vi "Remove Group IVI Devices.vi"(9 "IVI Names":string[][](array[string])=[["SNS_A", "SNS_A", "SRC_C", "SRC_C"], ["SNS_A", "SNS_A", "SRC_C", "SRC_C"], ["SNS_A", "SNS_A", "SRC_C", "SRC_C"], ["SNS_A", "SNS_A", "SRC_C", "SRC_C"], ["SNS_A", "SNS_A", "SRC_C", "SRC_C"], ["SNS_A", "SNS_A", "SRC_C", "SRC_C"], ["SNS_A", "SNS_A", "SRC_C", "SRC_C"], ["SNS_A", "SNS_A", "SRC_C", "SRC_C"], ["SNS_A", "SNS_A", "SRC_C", "SRC_C"], ["SNS_A", "SNS_A", "SRC_C", "SRC_C"], ["SNS_A", "SNS_A", "SRC_C", "SRC_C"], ["SNS_A", "SNS_A", "SRC_C", "SRC_C"], ["SNS_A", "SNS_A", "SRC_C", "SRC_C"], ["SNS_A", "SNS_A", "SRC_C", "SRC_C"], ["SNS_A", "SNS_A", "SRC_C", "SRC_C"], ["SNS_A", "SNS_A", "SRC_C", "SRC_C"], ["SNS_A", "SNS_A", "SRC_C", "SRC_C"], ["SNS_A", "SNS_A", "SRC_C", "SRC_C"], ["SNS_A", "SNS_A", "SRC_C", "SRC_C"], ["SNS_A", "SNS_A", "SRC_C", "SRC_C"], ["SNS_A", "SNS_A", "SRC_C", "SRC_C"], ["SNS_A", "SNS_A", "SRC_C", "SRC_C"], ["SNS_A", "SNS_A", "SRC_C", "SRC_C"], ["SNS_A", "SNS_A", "SRC_C", "SRC_C"], ["SNS_A", "SNS_A", "SRC_C", "SRC_C"], ["SNS_A", "SNS_A", "SRC_C", "SRC_C"], ["SNS_A", "SNS_A", "SRC_C", "SRC_C"], ["SNS_A", "SNS_A", "SRC_C", "SRC_C"], ["SNS_A", "SNS_A", "SRC_C", "SRC_C"], ["SNS_A", "SNS_A", "SRC_C", "SRC_C"], ["SNS_A", "SNS_A", "SRC_C", "SRC_C"], ["SNS_A", "SNS_A", "SRC_C", "SRC_C"], ["SNS_A", "SNS_A", "SRC_C", "SRC_C"], ["SNS_A", "SNS_A", "SRC_C", "SRC_C"], ["SNS_A", "SNS_A", "SRC_C", "SRC_C"], ["SNS_A", "SNS_A", "SRC_C", "SRC_C"], ["SNS_A", "SNS_A", "SRC_C", "SRC_C"], ["SNS_A", "SNS_A", "SRC_C", "SRC_C"], ["SNS_A", "SNS_A", "SRC_C", "SRC_C"], ["SNS_A", "SNS_A", "SRC_C", "SRC_C"], ["SNS_A", "SNS_A", "SRC_C", "SRC_C"], ["SNS_A", "SNS_A", "SRC_C", "SRC_C"], ["SNS_A", "SNS_A", "SRC_C", "SRC_C"], ["SNS_A", "SNS_A", "SRC_C", "SRC_C"], ["SNS_A", "SNS_A", "SRC_C", "SRC_C"], ["SNS_A", "SNS_A", "SRC_C", "SRC_C"], ["SNS_A", "SNS_A", "SRC_C", "SRC_C"], ["SNS_A", "SNS_A", "SRC_C", "SRC_C"], ["SNS_A", "SNS_A", "SRC_C", "SRC_C"], ["SNS_A", "SNS_A", "SRC_C", "SRC_C"], ["SNS_A", "SNS_A", "SRC_C", "SRC_C"], ["SNS_A", "SNS_A", "SRC_C", "SRC_C"], ["SNS_A", "SNS_A", "SRC_C", "SRC_C"], ["SNS_A", "SNS_A", "SRC_C", "SRC_C"], ["SNS_A", "SNS_A", "SRC_C", "SRC_C"], ["SNS_A", "SNS_A", "SRC_C", "SRC_C"], ["SNS_A", "SNS_A", "SRC_C", "SRC_C"], ["SNS_A", "SNS_A", "SRC_C", "SRC_C"], ["SNS_A", "SNS_A", "SRC_C", "SRC_C"], ["SNS_A", "SNS_A", "SRC_C", "SRC_C"], ["SNS_A", "SNS_A", "SRC_C", "SRC_C"], ["SNS_A", "SNS_A", "SRC_C", "SRC_C"], ["SNS_A", "SNS_A", "SRC_C", "SRC_C"], ["SNS_A", "SNS_A", "SRC_C", "SRC_C"], ["SNS_A", "SNS_A", "PXI1Slot14", ""], ["SNS_A", "SNS_A", "PXI1Slot14", ""], ["SNS_A", "SNS_A", "PXI1Slot14", ""], ["SNS_A", "SNS_A", "PXI1Slot14", ""], ["SNS_A", "SNS_A", "PXI1Slot14", ""], ["SNS_A", "SNS_A", "PXI1Slot14", ""], ["SNS_A", "SNS_A", "PXI1Slot14", ""], ["SNS_A", "SNS_A", "PXI1Slot14", ""], ["SNS_A", "SNS_A", "PXI1Slot14", ""], ["SNS_A", "SNS_A", "PXI1Slot14", ""], ["SNS_A", "SNS_A", "PXI1Slot14", ""], ["SNS_A", "SNS_A", "PXI1Slot14", ""], ["SNS_A", "SNS_A", "PXI1Slot14", ""], ["SNS_A", "SNS_A", "PXI1Slot14", ""], ["SNS_A", "SNS_A", "PXI1Slot14", ""], ["SNS_A", "SNS_A", "PXI1Slot14", ""], ["SNS_A", "SNS_A", "PXI1Slot14", ""], ["SNS_A", "SNS_A", "PXI1Slot14", ""], ["SNS_A", "SNS_A", "PXI1Slot14", ""], ["SNS_A", "SNS_A", "PXI1Slot14", ""], ["SNS_A", "SNS_A", "PXI1Slot14", ""], ["SNS_A", "SNS_A", "PXI1Slot14", ""], ["SNS_A", "SNS_A", "PXI1Slot14", ""], ["SNS_A", "SNS_A", "PXI1Slot14", ""], ["SNS_A", "SNS_A", "PXI1Slot14", ""], ["SNS_A", "SNS_A", "PXI1Slot14", ""], ["SNS_A", "SNS_A", "PXI1Slot14", ""], ["SNS_A", "SNS_A", "PXI1Slot14", ""], ["SNS_A", "SNS_A", "PXI1Slot14", ""], ["SNS_A", "SNS_A", "PXI1Slot14", ""], ["SNS_A", "SNS_A", "PXI1Slot14", ""], ["SNS_A", "SNS_A", "PXI1Slot14", ""], ["SNS_A", "SNS_A", "PXI1Slot14", ""], ["SNS_A", "SNS_A", "PXI1Slot14", ""], ["SNS_A", "SNS_A", "PXI1Slot14", ""], ["SNS_A", "SNS_A", "PXI1Slot14", ""], ["SNS_A", "SNS_A", "PXI1Slot14", ""], ["SNS_A", "SNS_A", "PXI1Slot14", ""], ["SNS_A", "SNS_A", "PXI1Slot14", ""], ["SNS_A", "SNS_A", "PXI1Slot14", ""], ["SNS_A", "SNS_A", "PXI1Slot14", ""], ["SNS_A", "SNS_A", "PXI1Slot14", ""], ["SNS_A", "SNS_A", "PXI1Slot14", ""], ["SNS_A", "SNS_A", "PXI1Slot14", ""], ["SNS_A", "SNS_A", "PXI1Slot14", ""], ["SNS_A", "SNS_A", "PXI1Slot14", ""], ["SNS_A", "SNS_A", "PXI1Slot14", ""], ["SNS_A", "SNS_A", "PXI1Slot14", ""], ["SNS_A", "SNS_A", "PXI1Slot14", ""], ["SNS_A", "SNS_A", "PXI1Slot14", ""], ["SNS_A", "SNS_A", "PXI1Slot14", ""], ["SNS_A", "SNS_A", "PXI1Slot14", ""], ["SNS_A", "SNS_A", "PXI1Slot14", ""], ["SNS_A", "SNS_A", "PXI1Slot14", ""], ["SNS_A", "SNS_A", "PXI1Slot14", ""], ["SNS_A", "SNS_A", "PXI1Slot14", ""], ["SNS_A", "SNS_A", "PXI1Slot14", ""], ["SNS_A", "SNS_A", "PXI1Slot14", ""], ["SNS_A", "SNS_A", "PXI1Slot14", ""], ["SNS_A", "SNS_A", "PXI1Slot14", ""], ["SNS_A", "SNS_A", "PXI1Slot14", ""], ["SNS_A", "SNS_A", "PXI1Slot14", ""], ["SNS_A", "SNS_A", "PXI1Slot14", ""]], 11 "Specifications":string[][](array[string])=[["Ch0", "[SNS_A/ab2->SNS_A/card1r2->SNS_A/c0]", "[SNS_A/ab3->SNS_A/card1r3->SNS_A/c1]", "[SRC_C/ab0->SRC_C/card1r0->SRC_C/c0]", "[SRC_C/ab1->SRC_C/card1r1->SRC_C/c1]"], ["Ch1", "[SNS_A/ab2->SNS_A/card1r2->SNS_A/c2]", "[SNS_A/ab3->SNS_A/card1r3->SNS_A/c3]", "[SRC_C/ab0->SRC_C/card1r0->SRC_C/c2]", "[SRC_C/ab1->SRC_C/card1r1->SRC_C/c3]"], ["Ch2", "[SNS_A/ab2->SNS_A/card1r2->SNS_A/c4]", "[SNS_A/ab3->SNS_A/card1r3->SNS_A/c5]", "[SRC_C/ab0->SRC_C/card1r0->SRC_C/c4]", "[SRC_C/ab1->SRC_C/card1r1->SRC_C/c5]"], ["Ch3", "[SNS_A/ab2->SNS_A/card1r2->SNS_A/c6]", "[SNS_A/ab3->SNS_A/card1r3->SNS_A/c7]", "[SRC_C/ab0->SRC_C/card1r0->SRC_C/c6]", "[SRC_C/ab1->SRC_C/card1r1->SRC_C/c7]"], ["Ch4", "[SNS_A/ab2->SNS_A/card1r2->SNS_A/c8]", "[SNS_A/ab3->SNS_A/card1r3->SNS_A/c9]", "[SRC_C/ab0->SRC_C/card1r0->SRC_C/c8]", "[SRC_C/ab1->SRC_C/card1r1->SRC_C/c9]"], ["Ch5", "[SNS_A/ab2->SNS_A/card1r2->SNS_A/c10]", "[SNS_A/ab3->SNS_A/card1r3->SNS_A/c11]", "[SRC_C/ab0->SRC_C/card1r0->SRC_C/c10]", "[SRC_C/ab1->SRC_C/card1r1->SRC_C/c11]"], ["Ch6", "[SNS_A/ab2->SNS_A/card1r2->SNS_A/c12]", "[SNS_A/ab3->SNS_A/card1r3->SNS_A/c13]", "[SRC_C/ab0->SRC_C/card1r0->SRC_C/c12]", "[SRC_C/ab1->SRC_C/card1r1->SRC_C/c13]"], ["Ch7", "[SNS_A/ab2->SNS_A/card1r2->SNS_A/c14]", "[SNS_A/ab3->SNS_A/card1r3->SNS_A/c15]", "[SRC_C/ab0->SRC_C/card1r0->SRC_C/c14]", "[SRC_C/ab1->SRC_C/card1r1->SRC_C/c15]"], ["Ch8", "[SNS_A/ab2->SNS_A/card1r2->SNS_A/c16]", "[SNS_A/ab3->SNS_A/card1r3->SNS_A/c17]", "[SRC_C/ab0->SRC_C/card1r0->SRC_C/c16]", "[SRC_C/ab1->SRC_C/card1r1->SRC_C/c17]"], ["Ch9", "[SNS_A/ab2->SNS_A/card1r2->SNS_A/c18]", "[SNS_A/ab3->SNS_A/card1r3->SNS_A/c19]", "[SRC_C/ab0->SRC_C/card1r0->SRC_C/c18]", "[SRC_C/ab1->SRC_C/card1r1->SRC_C/c19]"], ["Ch10", "[SNS_A/ab2->SNS_A/card1r2->SNS_A/c20]", "[SNS_A/ab3->SNS_A/card1r3->SNS_A/c21]", "[SRC_C/ab0->SRC_C/card1r0->SRC_C/c20]", "[SRC_C/ab1->SRC_C/card1r1->SRC_C/c21]"], ["Ch11", "[SNS_A/ab2->SNS_A/card1r2->SNS_A/c22]", "[SNS_A/ab3->SNS_A/card1r3->SNS_A/c23]", "[SRC_C/ab0->SRC_C/card1r0->SRC_C/c22]", "[SRC_C/ab1->SRC_C/card1r1->SRC_C/c23]"], ["Ch12", "[SNS_A/ab2->SNS_A/card1r2->SNS_A/c24]", "[SNS_A/ab3->SNS_A/card1r3->SNS_A/c25]", "[SRC_C/ab0->SRC_C/card1r0->SRC_C/c24]", "[SRC_C/ab1->SRC_C/card1r1->SRC_C/c25]"], ["Ch13", "[SNS_A/ab2->SNS_A/card1r2->SNS_A/c26]", "[SNS_A/ab3->SNS_A/card1r3->SNS_A/c27]", "[SRC_C/ab0->SRC_C/card1r0->SRC_C/c26]", "[SRC_C/ab1->SRC_C/card1r1->SRC_C/c27]"], ["Ch14", "[SNS_A/ab2->SNS_A/card1r2->SNS_A/c28]", "[SNS_A/ab3->SNS_A/card1r3->SNS_A/c29]", "[SRC_C/ab0->SRC_C/card1r0->SRC_C/c28]", "[SRC_C/ab1->SRC_C/card1r1->SRC_C/c29]"], ["Ch15", "[SNS_A/ab2->SNS_A/card1r2->SNS_A/c30]", "[SNS_A/ab3->SNS_A/card1r3->SNS_A/c31]", "[SRC_C/ab0->SRC_C/card1r0->SRC_C/c30]", "[SRC_C/ab1->SRC_C/card1r1->SRC_C/c31]"], ["Ch16", "[SNS_A/ab2->SNS_A/card1r2->SNS_A/c32]", "[SNS_A/ab3->SNS_A/card1r3->SNS_A/c33]", "[SRC_C/ab0->SRC_C/card1r0->SRC_C/c32]", "[SRC_C/ab1->SRC_C/card1r1->SRC_C/c33]"], ["Ch17", "[SNS_A/ab2->SNS_A/card1r2->SNS_A/c34]", "[SNS_A/ab3->SNS_A/card1r3->SNS_A/c35]", "[SRC_C/ab0->SRC_C/card1r0->SRC_C/c34]", "[SRC_C/ab1->SRC_C/card1r1->SRC_C/c35]"], ["Ch18", "[SNS_A/ab2->SNS_A/card1r2->SNS_A/c36]", "[SNS_A/ab3->SNS_A/card1r3->SNS_A/c37]", "[SRC_C/ab0->SRC_C/card1r0->SRC_C/c36]", "[SRC_C/ab1->SRC_C/card1r1->SRC_C/c37]"], ["Ch19", "[SNS_A/ab2->SNS_A/card1r2->SNS_A/c38]", "[SNS_A/ab3->SNS_A/card1r3->SNS_A/c39]", "[SRC_C/ab0->SRC_C/card1r0->SRC_C/c38]", "[SRC_C/ab1->SRC_C/card1r1->SRC_C/c39]"], ["Ch20", "[SNS_A/ab2->SNS_A/card1r2->SNS_A/c40]", "[SNS_A/ab3->SNS_A/card1r3->SNS_A/c41]", "[SRC_C/ab0->SRC_C/card1r0->SRC_C/c40]", "[SRC_C/ab1->SRC_C/card1r1->SRC_C/c41]"], ["Ch21", "[SNS_A/ab2->SNS_A/card1r2->SNS_A/c42]", "[SNS_A/ab3->SNS_A/card2r3->SNS_A/c43]", "[SRC_C/ab0->SRC_C/card1r0->SRC_C/c42]", "[SRC_C/ab1->SRC_C/card2r1->SRC_C/c43]"], ["Ch22", "[SNS_A/ab2->SNS_A/card2r2->SNS_A/c44]", "[SNS_A/ab3->SNS_A/card2r3->SNS_A/c45]", "[SRC_C/ab0->SRC_C/card2r0->SRC_C/c44]", "[SRC_C/ab1->SRC_C/card2r1->SRC_C/c45]"], ["Ch23", "[SNS_A/ab2->SNS_A/card2r2->SNS_A/c46]", "[SNS_A/ab3->SNS_A/card2r3->SNS_A/c47]", "[SRC_C/ab0->SRC_C/card2r0->SRC_C/c46]", "[SRC_C/ab1->SRC_C/card2r1->SRC_C/c47]"], ["Ch24", "[SNS_A/ab2->SNS_A/card2r2->SNS_A/c48]", "[SNS_A/ab3->SNS_A/card2r3->SNS_A/c49]", "[SRC_C/ab0->SRC_C/card2r0->SRC_C/c48]", "[SRC_C/ab1->SRC_C/card2r1->SRC_C/c49]"], ["Ch25", "[SNS_A/ab2->SNS_A/card2r2->SNS_A/c50]", "[SNS_A/ab3->SNS_A/card2r3->SNS_A/c51]", "[SRC_C/ab0->SRC_C/card2r0->SRC_C/c50]", "[SRC_C/ab1->SRC_C/card2r1->SRC_C/c51]"], ["Ch26", "[SNS_A/ab2->SNS_A/card2r2->SNS_A/c52]", "[SNS_A/ab3->SNS_A/card2r3->SNS_A/c53]", "[SRC_C/ab0->SRC_C/card2r0->SRC_C/c52]", "[SRC_C/ab1->SRC_C/card2r1->SRC_C/c53]"], ["Ch27", "[SNS_A/ab2->SNS_A/card2r2->SNS_A/c54]", "[SNS_A/ab3->SNS_A/card2r3->SNS_A/c55]", "[SRC_C/ab0->SRC_C/card2r0->SRC_C/c54]", "[SRC_C/ab1->SRC_C/card2r1->SRC_C/c55]"], ["Ch28", "[SNS_A/ab2->SNS_A/card2r2->SNS_A/c56]", "[SNS_A/ab3->SNS_A/card2r3->SNS_A/c57]", "[SRC_C/ab0->SRC_C/card2r0->SRC_C/c56]", "[SRC_C/ab1->SRC_C/card2r1->SRC_C/c57]"], ["Ch29", "[SNS_A/ab2->SNS_A/card2r2->SNS_A/c58]", "[SNS_A/ab3->SNS_A/card2r3->SNS_A/c59]", "[SRC_C/ab0->SRC_C/card2r0->SRC_C/c58]", "[SRC_C/ab1->SRC_C/card2r1->SRC_C/c59]"], ["Ch30", "[SNS_A/ab2->SNS_A/card2r2->SNS_A/c60]", "[SNS_A/ab3->SNS_A/card2r3->SNS_A/c61]", "[SRC_C/ab0->SRC_C/card2r0->SRC_C/c60]", "[SRC_C/ab1->SRC_C/card2r1->SRC_C/c61]"], ["Ch31", "[SNS_A/ab2->SNS_A/card2r2->SNS_A/c62]", "[SNS_A/ab3->SNS_A/card2r3->SNS_A/c63]", "[SRC_C/ab0->SRC_C/card2r0->SRC_C/c62]", "[SRC_C/ab1->SRC_C/card2r1->SRC_C/c63]"], ["Ch32", "[SNS_A/ab2->SNS_A/card2r2->SNS_A/c64]", "[SNS_A/ab3->SNS_A/card2r3->SNS_A/c65]", "[SRC_C/ab0->SRC_C/card2r0->SRC_C/c64]", "[SRC_C/ab1->SRC_C/card2r1->SRC_C/c65]"], ["Ch33", "[SNS_A/ab2->SNS_A/card2r2->SNS_A/c66]", "[SNS_A/ab3->SNS_A/card2r3->SNS_A/c67]", "[SRC_C/ab0->SRC_C/card2r0->SRC_C/c66]", "[SRC_C/ab1->SRC_C/card2r1->SRC_C/c67]"], ["Ch34", "[SNS_A/ab2->SNS_A/card2r2->SNS_A/c68]", "[SNS_A/ab3->SNS_A/card2r3->SNS_A/c69]", "[SRC_C/ab0->SRC_C/card2r0->SRC_C/c68]", "[SRC_C/ab1->SRC_C/card2r1->SRC_C/c69]"], ["Ch35", "[SNS_A/ab2->SNS_A/card2r2->SNS_A/c70]", "[SNS_A/ab3->SNS_A/card2r3->SNS_A/c71]", "[SRC_C/ab0->SRC_C/card2r0->SRC_C/c70]", "[SRC_C/ab1->SRC_C/card2r1->SRC_C/c71]"], ["Ch36", "[SNS_A/ab2->SNS_A/card2r2->SNS_A/c72]", "[SNS_A/ab3->SNS_A/card2r3->SNS_A/c73]", "[SRC_C/ab0->SRC_C/card2r0->SRC_C/c72]", "[SRC_C/ab1->SRC_C/card2r1->SRC_C/c73]"], ["Ch37", "[SNS_A/ab2->SNS_A/card2r2->SNS_A/c74]", "[SNS_A/ab3->SNS_A/card2r3->SNS_A/c75]", "[SRC_C/ab0->SRC_C/card2r0->SRC_C/c74]", "[SRC_C/ab1->SRC_C/card2r1->SRC_C/c75]"], ["Ch38", "[SNS_A/ab2->SNS_A/card2r2->SNS_A/c76]", "[SNS_A/ab3->SNS_A/card2r3->SNS_A/c77]", "[SRC_C/ab0->SRC_C/card2r0->SRC_C/c76]", "[SRC_C/ab1->SRC_C/card2r1->SRC_C/c77]"], ["Ch39", "[SNS_A/ab2->SNS_A/card2r2->SNS_A/c78]", "[SNS_A/ab3->SNS_A/card2r3->SNS_A/c79]", "[SRC_C/ab0->SRC_C/card2r0->SRC_C/c78]", "[SRC_C/ab1->SRC_C/card2r1->SRC_C/c79]"], ["Ch40", "[SNS_A/ab2->SNS_A/card2r2->SNS_A/c80]", "[SNS_A/ab3->SNS_A/card2r3->SNS_A/c81]", "[SRC_C/ab0->SRC_C/card2r0->SRC_C/c80]", "[SRC_C/ab1->SRC_C/card2r1->SRC_C/c81]"], ["Ch41", "[SNS_A/ab2->SNS_A/card2r2->SNS_A/c82]", "[SNS_A/ab3->SNS_A/card2r3->SNS_A/c83]", "[SRC_C/ab0->SRC_C/card2r0->SRC_C/c82]", "[SRC_C/ab1->SRC_C/card2r1->SRC_C/c83]"], ["Ch42", "[SNS_A/ab2->SNS_A/card2r2->SNS_A/c84]", "[SNS_A/ab3->SNS_A/card2r3->SNS_A/c85]", "[SRC_C/ab0->SRC_C/card2r0->SRC_C/c84]", "[SRC_C/ab1->SRC_C/card2r1->SRC_C/c85]"], ["Ch43", "[SNS_A/ab2->SNS_A/card3r2->SNS_A/c86]", "[SNS_A/ab3->SNS_A/card3r3->SNS_A/c87]", "[SRC_C/ab0->SRC_C/card3r0->SRC_C/c86]", "[SRC_C/ab1->SRC_C/card3r1->SRC_C/c87]"], ["Ch44", "[SNS_A/ab2->SNS_A/card3r2->SNS_A/c88]", "[SNS_A/ab3->SNS_A/card3r3->SNS_A/c89]", "[SRC_C/ab0->SRC_C/card3r0->SRC_C/c88]", "[SRC_C/ab1->SRC_C/card3r1->SRC_C/c89]"], ["Ch45", "[SNS_A/ab2->SNS_A/card3r2->SNS_A/c90]", "[SNS_A/ab3->SNS_A/card3r3->SNS_A/c91]", "[SRC_C/ab0->SRC_C/card3r0->SRC_C/c90]", "[SRC_C/ab1->SRC_C/card3r1->SRC_C/c91]"], ["Ch46", "[SNS_A/ab2->SNS_A/card3r2->SNS_A/c92]", "[SNS_A/ab3->SNS_A/card3r3->SNS_A/c93]", "[SRC_C/ab0->SRC_C/card3r0->SRC_C/c92]", "[SRC_C/ab1->SRC_C/card3r1->SRC_C/c93]"], ["Ch47", "[SNS_A/ab2->SNS_A/card3r2->SNS_A/c94]", "[SNS_A/ab3->SNS_A/card3r3->SNS_A/c95]", "[SRC_C/ab0->SRC_C/card3r0->SRC_C/c94]", "[SRC_C/ab1->SRC_C/card3r1->SRC_C/c95]"], ["Ch48", "[SNS_A/ab2->SNS_A/card3r2->SNS_A/c96]", "[SNS_A/ab3->SNS_A/card3r3->SNS_A/c97]", "[SRC_C/ab0->SRC_C/card3r0->SRC_C/c96]", "[SRC_C/ab1->SRC_C/card3r1->SRC_C/c97]"], ["Ch49", "[SNS_A/ab2->SNS_A/card3r2->SNS_A/c98]", "[SNS_A/ab3->SNS_A/card3r3->SNS_A/c99]", "[SRC_C/ab0->SRC_C/card3r0->SRC_C/c98]", "[SRC_C/ab1->SRC_C/card3r1->SRC_C/c99]"], ["Ch50", "[SNS_A/ab2->SNS_A/card3r2->SNS_A/c100]", "[SNS_A/ab3->SNS_A/card3r3->SNS_A/c101]", "[SRC_C/ab0->SRC_C/card3r0->SRC_C/c100]", "[SRC_C/ab1->SRC_C/card3r1->SRC_C/c101]"], ["Ch51", "[SNS_A/ab2->SNS_A/card3r2->SNS_A/c102]", "[SNS_A/ab3->SNS_A/card3r3->SNS_A/c103]", "[SRC_C/ab0->SRC_C/card3r0->SRC_C/c102]", "[SRC_C/ab1->SRC_C/card3r1->SRC_C/c103]"], ["Ch52", "[SNS_A/ab2->SNS_A/card3r2->SNS_A/c104]", "[SNS_A/ab3->SNS_A/card3r3->SNS_A/c105]", "[SRC_C/ab0->SRC_C/card3r0->SRC_C/c104]", "[SRC_C/ab1->SRC_C/card3r1->SRC_C/c105]"], ["Ch53", "[SNS_A/ab2->SNS_A/card3r2->SNS_A/c106]", "[SNS_A/ab3->SNS_A/card3r3->SNS_A/c107]", "[SRC_C/ab0->SRC_C/card3r0->SRC_C/c106]", "[SRC_C/ab1->SRC_C/card3r1->SRC_C/c107]"], ["Ch54", "[SNS_A/ab2->SNS_A/card3r2->SNS_A/c108]", "[SNS_A/ab3->SNS_A/card3r3->SNS_A/c109]", "[SRC_C/ab0->SRC_C/card3r0->SRC_C/c108]", "[SRC_C/ab1->SRC_C/card3r1->SRC_C/c109]"], ["Ch55", "[SNS_A/ab2->SNS_A/card3r2->SNS_A/c110]", "[SNS_A/ab3->SNS_A/card3r3->SNS_A/c111]", "[SRC_C/ab0->SRC_C/card3r0->SRC_C/c110]", "[SRC_C/ab1->SRC_C/card3r1->SRC_C/c111]"], ["Ch56", "[SNS_A/ab2->SNS_A/card3r2->SNS_A/c112]", "[SNS_A/ab3->SNS_A/card3r3->SNS_A/c113]", "[SRC_C/ab0->SRC_C/card3r0->SRC_C/c112]", "[SRC_C/ab1->SRC_C/card3r1->SRC_C/c113]"], ["Ch57", "[SNS_A/ab2->SNS_A/card3r2->SNS_A/c114]", "[SNS_A/ab3->SNS_A/card3r3->SNS_A/c115]", "[SRC_C/ab0->SRC_C/card3r0->SRC_C/c114]", "[SRC_C/ab1->SRC_C/card3r1->SRC_C/c115]"], ["Ch58", "[SNS_A/ab2->SNS_A/card3r2->SNS_A/c116]", "[SNS_A/ab3->SNS_A/card3r3->SNS_A/c117]", "[SRC_C/ab0->SRC_C/card3r0->SRC_C/c116]", "[SRC_C/ab1->SRC_C/card3r1->SRC_C/c117]"], ["Ch59", "[SNS_A/ab2->SNS_A/card3r2->SNS_A/c118]", "[SNS_A/ab3->SNS_A/card3r3->SNS_A/c119]", "[SRC_C/ab0->SRC_C/card3r0->SRC_C/c118]", "[SRC_C/ab1->SRC_C/card3r1->SRC_C/c119]"], ["Ch60", "[SNS_A/ab2->SNS_A/card3r2->SNS_A/c120]", "[SNS_A/ab3->SNS_A/card3r3->SNS_A/c121]", "[SRC_C/ab0->SRC_C/card3r0->SRC_C/c120]", "[SRC_C/ab1->SRC_C/card3r1->SRC_C/c121]"], ["Ch61", "[SNS_A/ab2->SNS_A/card3r2->SNS_A/c122]", "[SNS_A/ab3->SNS_A/card3r3->SNS_A/c123]", "[SRC_C/ab0->SRC_C/card3r0->SRC_C/c122]", "[SRC_C/ab1->SRC_C/card3r1->SRC_C/c123]"], ["Ch62", "[SNS_A/ab2->SNS_A/card3r2->SNS_A/c124]", "[SNS_A/ab3->SNS_A/card3r3->SNS_A/c125]", "[SRC_C/ab0->SRC_C/card3r0->SRC_C/c124]", "[SRC_C/ab1->SRC_C/card3r1->SRC_C/c125]"], ["Ch63", "[SNS_A/ab2->SNS_A/card3r2->SNS_A/c126]", "[SNS_A/ab3->SNS_A/card3r3->SNS_A/c127]", "[SRC_C/ab0->SRC_C/card3r0->SRC_C/c126]", "[SRC_C/ab1->SRC_C/card3r1->SRC_C/c127]"], ["Ch64", "[SNS_A/ab2->SNS_A/card3r2->SNS_A/c128]", "[SNS_A/ab3->SNS_A/card4r3->SNS_A/c129]", "[PXI1Slot14/ch0->PXI1Slot14/com]", ""], ["Ch65", "[SNS_A/ab2->SNS_A/card4r2->SNS_A/c130]", "[SNS_A/ab3->SNS_A/card4r3->SNS_A/c131]", "[PXI1Slot14/ch1->PXI1Slot14/com]", ""], ["Ch66", "[SNS_A/ab2->SNS_A/card4r2->SNS_A/c132]", "[SNS_A/ab3->SNS_A/card4r3->SNS_A/c133]", "[PXI1Slot14/ch2->PXI1Slot14/com]", ""], ["Ch67", "[SNS_A/ab2->SNS_A/card4r2->SNS_A/c134]", "[SNS_A/ab3->SNS_A/card4r3->SNS_A/c135]", "[PXI1Slot14/ch3->PXI1Slot14/com]", ""], ["Ch68", "[SNS_A/ab2->SNS_A/card4r2->SNS_A/c136]", "[SNS_A/ab3->SNS_A/card4r3->SNS_A/c137]", "[PXI1Slot14/ch4->PXI1Slot14/com]", ""], ["Ch69", "[SNS_A/ab2->SNS_A/card4r2->SNS_A/c138]", "[SNS_A/ab3->SNS_A/card4r3->SNS_A/c139]", "[PXI1Slot14/ch5->PXI1Slot14/com]", ""], ["Ch70", "[SNS_A/ab2->SNS_A/card4r2->SNS_A/c140]", "[SNS_A/ab3->SNS_A/card4r3->SNS_A/c141]", "[PXI1Slot14/ch6->PXI1Slot14/com]", ""], ["Ch71", "[SNS_A/ab2->SNS_A/card4r2->SNS_A/c142]", "[SNS_A/ab3->SNS_A/card4r3->SNS_A/c143]", "[PXI1Slot14/ch7->PXI1Slot14/com]", ""], ["Ch72", "[SNS_A/ab2->SNS_A/card4r2->SNS_A/c144]", "[SNS_A/ab3->SNS_A/card4r3->SNS_A/c145]", "[PXI1Slot14/ch8->PXI1Slot14/com]", ""], ["Ch73", "[SNS_A/ab2->SNS_A/card4r2->SNS_A/c146]", "[SNS_A/ab3->SNS_A/card4r3->SNS_A/c147]", "[PXI1Slot14/ch9->PXI1Slot14/com]", ""], ["Ch74", "[SNS_A/ab2->SNS_A/card4r2->SNS_A/c148]", "[SNS_A/ab3->SNS_A/card4r3->SNS_A/c149]", "[PXI1Slot14/ch10->PXI1Slot14/com]", ""], ["Ch75", "[SNS_A/ab2->SNS_A/card4r2->SNS_A/c150]", "[SNS_A/ab3->SNS_A/card4r3->SNS_A/c151]", "[PXI1Slot14/ch11->PXI1Slot14/com]", ""], ["Ch76", "[SNS_A/ab2->SNS_A/card4r2->SNS_A/c152]", "[SNS_A/ab3->SNS_A/card4r3->SNS_A/c153]", "[PXI1Slot14/ch12->PXI1Slot14/com]", ""], ["Ch77", "[SNS_A/ab2->SNS_A/card4r2->SNS_A/c154]", "[SNS_A/ab3->SNS_A/card4r3->SNS_A/c155]", "[PXI1Slot14/ch13->PXI1Slot14/com]", ""], ["Ch78", "[SNS_A/ab2->SNS_A/card4r2->SNS_A/c156]", "[SNS_A/ab3->SNS_A/card4r3->SNS_A/c157]", "[PXI1Slot14/ch14->PXI1Slot14/com]", ""], ["Ch79", "[SNS_A/ab2->SNS_A/card4r2->SNS_A/c158]", "[SNS_A/ab3->SNS_A/card4r3->SNS_A/c159]", "[PXI1Slot14/ch15->PXI1Slot14/com]", ""], ["Ch80", "[SNS_A/ab2->SNS_A/card4r2->SNS_A/c160]", "[SNS_A/ab3->SNS_A/card4r3->SNS_A/c161]", "[PXI1Slot14/ch16->PXI1Slot14/com]", ""], ["Ch81", "[SNS_A/ab2->SNS_A/card4r2->SNS_A/c162]", "[SNS_A/ab3->SNS_A/card4r3->SNS_A/c163]", "[PXI1Slot14/ch17->PXI1Slot14/com]", ""], ["Ch82", "[SNS_A/ab2->SNS_A/card4r2->SNS_A/c164]", "[SNS_A/ab3->SNS_A/card4r3->SNS_A/c165]", "[PXI1Slot14/ch18->PXI1Slot14/com]", ""], ["Ch83", "[SNS_A/ab2->SNS_A/card4r2->SNS_A/c166]", "[SNS_A/ab3->SNS_A/card4r3->SNS_A/c167]", "[PXI1Slot14/ch19->PXI1Slot14/com]", ""], ["Ch84", "[SNS_A/ab2->SNS_A/card4r2->SNS_A/c168]", "[SNS_A/ab3->SNS_A/card4r3->SNS_A/c169]", "[PXI1Slot14/ch20->PXI1Slot14/com]", ""], ["Ch85", "[SNS_A/ab2->SNS_A/card4r2->SNS_A/c170]", "[SNS_A/ab3->SNS_A/card4r3->SNS_A/c171]", "[PXI1Slot14/ch21->PXI1Slot14/com]", ""], ["Ch86", "[SNS_A/ab2->SNS_A/card5r2->SNS_A/c172]", "[SNS_A/ab3->SNS_A/card5r3->SNS_A/c173]", "[PXI1Slot14/ch22->PXI1Slot14/com]", ""], ["Ch87", "[SNS_A/ab2->SNS_A/card5r2->SNS_A/c174]", "[SNS_A/ab3->SNS_A/card5r3->SNS_A/c175]", "[PXI1Slot14/ch23->PXI1Slot14/com]", ""], ["Ch88", "[SNS_A/ab2->SNS_A/card5r2->SNS_A/c176]", "[SNS_A/ab3->SNS_A/card5r3->SNS_A/c177]", "[PXI1Slot14/ch24->PXI1Slot14/com]", ""], ["Ch89", "[SNS_A/ab2->SNS_A/card5r2->SNS_A/c178]", "[SNS_A/ab3->SNS_A/card5r3->SNS_A/c179]", "[PXI1Slot14/ch25->PXI1Slot14/com]", ""], ["Ch90", "[SNS_A/ab2->SNS_A/card5r2->SNS_A/c180]", "[SNS_A/ab3->SNS_A/card5r3->SNS_A/c181]", "[PXI1Slot14/ch26->PXI1Slot14/com]", ""], ["Ch91", "[SNS_A/ab2->SNS_A/card5r2->SNS_A/c182]", "[SNS_A/ab3->SNS_A/card5r3->SNS_A/c183]", "[PXI1Slot14/ch27->PXI1Slot14/com]", ""], ["Ch92", "[SNS_A/ab2->SNS_A/card5r2->SNS_A/c184]", "[SNS_A/ab3->SNS_A/card5r3->SNS_A/c185]", "[PXI1Slot14/ch28->PXI1Slot14/com]", ""], ["Ch93", "[SNS_A/ab2->SNS_A/card5r2->SNS_A/c186]", "[SNS_A/ab3->SNS_A/card5r3->SNS_A/c187]", "[PXI1Slot14/ch29->PXI1Slot14/com]", ""], ["Ch94", "[SNS_A/ab2->SNS_A/card5r2->SNS_A/c188]", "[SNS_A/ab3->SNS_A/card5r3->SNS_A/c189]", "[PXI1Slot14/ch30->PXI1Slot14/com]", ""], ["Ch95", "[SNS_A/ab2->SNS_A/card5r2->SNS_A/c190]", "[SNS_A/ab3->SNS_A/card5r3->SNS_A/c191]", "[PXI1Slot14/ch31->PXI1Slot14/com]", ""], ["Ch96", "[SNS_A/ab2->SNS_A/card5r2->SNS_A/c192]", "[SNS_A/ab3->SNS_A/card5r3->SNS_A/c193]", "[PXI1Slot14/ch32->PXI1Slot14/com]", ""], ["Ch97", "[SNS_A/ab2->SNS_A/card5r2->SNS_A/c194]", "[SNS_A/ab3->SNS_A/card5r3->SNS_A/c195]", "[PXI1Slot14/ch33->PXI1Slot14/com]", ""], ["Ch98", "[SNS_A/ab2->SNS_A/card5r2->SNS_A/c196]", "[SNS_A/ab3->SNS_A/card5r3->SNS_A/c197]", "[PXI1Slot14/ch34->PXI1Slot14/com]", ""], ["Ch99", "[SNS_A/ab2->SNS_A/card5r2->SNS_A/c198]", "[SNS_A/ab3->SNS_A/card5r3->SNS_A/c199]", "[PXI1Slot14/ch35->PXI1Slot14/com]", ""], ["Ch100", "[SNS_A/ab2->SNS_A/card5r2->SNS_A/c200]", "[SNS_A/ab3->SNS_A/card5r3->SNS_A/c201]", "[PXI1Slot14/ch36->PXI1Slot14/com]", ""], ["Ch101", "[SNS_A/ab2->SNS_A/card5r2->SNS_A/c202]", "[SNS_A/ab3->SNS_A/card5r3->SNS_A/c203]", "[PXI1Slot14/ch37->PXI1Slot14/com]", ""], ["Ch102", "[SNS_A/ab2->SNS_A/card5r2->SNS_A/c204]", "[SNS_A/ab3->SNS_A/card5r3->SNS_A/c205]", "[PXI1Slot14/ch38->PXI1Slot14/com]", ""], ["Ch103", "[SNS_A/ab2->SNS_A/card5r2->SNS_A/c206]", "[SNS_A/ab3->SNS_A/card5r3->SNS_A/c207]", "[PXI1Slot14/ch39->PXI1Slot14/com]", ""], ["Ch104", "[SNS_A/ab2->SNS_A/card5r2->SNS_A/c208]", "[SNS_A/ab3->SNS_A/card5r3->SNS_A/c209]", "[PXI1Slot14/ch40->PXI1Slot14/com]", ""], ["Ch105", "[SNS_A/ab2->SNS_A/card5r2->SNS_A/c210]", "[SNS_A/ab3->SNS_A/card5r3->SNS_A/c211]", "[PXI1Slot14/ch41->PXI1Slot14/com]", ""], ["Ch106", "[SNS_A/ab2->SNS_A/card5r2->SNS_A/c212]", "[SNS_A/ab3->SNS_A/card5r3->SNS_A/c213]", "[PXI1Slot14/ch42->PXI1Slot14/com]", ""], ["Ch107", "[SNS_A/ab2->SNS_A/card5r2->SNS_A/c214]", "[SNS_A/ab3->SNS_A/card6r3->SNS_A/c215]", "[PXI1Slot14/ch43->PXI1Slot14/com]", ""], ["Ch108", "[SNS_A/ab2->SNS_A/card6r2->SNS_A/c216]", "[SNS_A/ab3->SNS_A/card6r3->SNS_A/c217]", "[PXI1Slot14/ch44->PXI1Slot14/com]", ""], ["Ch109", "[SNS_A/ab2->SNS_A/card6r2->SNS_A/c218]", "[SNS_A/ab3->SNS_A/card6r3->SNS_A/c219]", "[PXI1Slot14/ch45->PXI1Slot14/com]", ""], ["Ch110", "[SNS_A/ab2->SNS_A/card6r2->SNS_A/c220]", "[SNS_A/ab3->SNS_A/card6r3->SNS_A/c221]", "[PXI1Slot14/ch46->PXI1Slot14/com]", ""], ["Ch111", "[SNS_A/ab2->SNS_A/card6r2->SNS_A/c222]", "[SNS_A/ab3->SNS_A/card6r3->SNS_A/c223]", "[PXI1Slot14/ch47->PXI1Slot14/com]", ""], ["Ch112", "[SNS_A/ab2->SNS_A/card6r2->SNS_A/c224]", "[SNS_A/ab3->SNS_A/card6r3->SNS_A/c225]", "[PXI1Slot14/ch48->PXI1Slot14/com]", ""], ["Ch113", "[SNS_A/ab2->SNS_A/card6r2->SNS_A/c226]", "[SNS_A/ab3->SNS_A/card6r3->SNS_A/c227]", "[PXI1Slot14/ch49->PXI1Slot14/com]", ""], ["Ch114", "[SNS_A/ab2->SNS_A/card6r2->SNS_A/c228]", "[SNS_A/ab3->SNS_A/card6r3->SNS_A/c229]", "[PXI1Slot14/ch50->PXI1Slot14/com]", ""], ["Ch115", "[SNS_A/ab2->SNS_A/card6r2->SNS_A/c230]", "[SNS_A/ab3->SNS_A/card6r3->SNS_A/c231]", "[PXI1Slot14/ch51->PXI1Slot14/com]", ""], ["Ch116", "[SNS_A/ab2->SNS_A/card6r2->SNS_A/c232]", "[SNS_A/ab3->SNS_A/card6r3->SNS_A/c233]", "[PXI1Slot14/ch52->PXI1Slot14/com]", ""], ["Ch117", "[SNS_A/ab2->SNS_A/card6r2->SNS_A/c234]", "[SNS_A/ab3->SNS_A/card6r3->SNS_A/c235]", "[PXI1Slot14/ch53->PXI1Slot14/com]", ""], ["Ch118", "[SNS_A/ab2->SNS_A/card6r2->SNS_A/c236]", "[SNS_A/ab3->SNS_A/card6r3->SNS_A/c237]", "[PXI1Slot14/ch54->PXI1Slot14/com]", ""], ["Ch119", "[SNS_A/ab2->SNS_A/card6r2->SNS_A/c238]", "[SNS_A/ab3->SNS_A/card6r3->SNS_A/c239]", "[PXI1Slot14/ch55->PXI1Slot14/com]", ""], ["Ch120", "[SNS_A/ab2->SNS_A/card6r2->SNS_A/c240]", "[SNS_A/ab3->SNS_A/card6r3->SNS_A/c241]", "[PXI1Slot14/ch56->PXI1Slot14/com]", ""], ["Ch121", "[SNS_A/ab2->SNS_A/card6r2->SNS_A/c242]", "[SNS_A/ab3->SNS_A/card6r3->SNS_A/c243]", "[PXI1Slot14/ch57->PXI1Slot14/com]", ""], ["Ch122", "[SNS_A/ab2->SNS_A/card6r2->SNS_A/c244]", "[SNS_A/ab3->SNS_A/card6r3->SNS_A/c245]", "[PXI1Slot14/ch58->PXI1Slot14/com]", ""], ["Ch123", "[SNS_A/ab2->SNS_A/card6r2->SNS_A/c246]", "[SNS_A/ab3->SNS_A/card6r3->SNS_A/c247]", "[PXI1Slot14/ch59->PXI1Slot14/com]", ""], ["Ch124", "[SNS_A/ab2->SNS_A/card6r2->SNS_A/c248]", "[SNS_A/ab3->SNS_A/card6r3->SNS_A/c249]", "[PXI1Slot14/ch60->PXI1Slot14/com]", ""], ["Ch125", "[SNS_A/ab2->SNS_A/card6r2->SNS_A/c250]", "[SNS_A/ab3->SNS_A/card6r3->SNS_A/c251]", "[PXI1Slot14/ch61->PXI1Slot14/com]", ""], ["Ch126", "[SNS_A/ab2->SNS_A/card6r2->SNS_A/c252]", "[SNS_A/ab3->SNS_A/card6r3->SNS_A/c253]", "[PXI1Slot14/ch62->PXI1Slot14/com]", ""]]) -> (1 "Route Specs":string[][](array[string]))   [LabVIEW 2019]
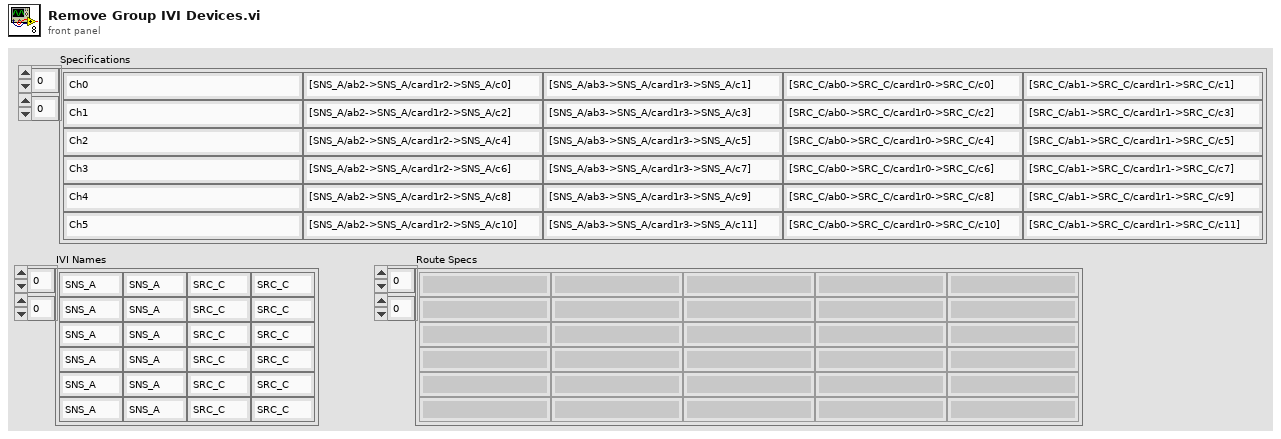
[diagram p1: front panel]
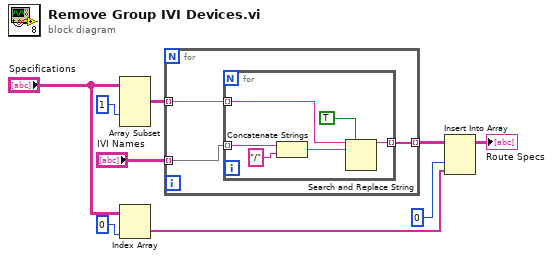
[diagram p0: block diagram]
diagram:
  n1 = Array Subset(array="Specifications", index (col)=1 ("index")) -> (w7:string[][])  [unwired: 3 in]
  n2 = Index Array(array="Specifications", index (col)=0 ("disabled index (col)")) -> (element=w2:string[])  [unwired: 1 in]
  n3 = for {
    tunnel: "IVI Names" -> [w12] mode=indexing
    tunnel: w7 -> [w11] mode=indexing
    tunnel: [w10] -> w4 mode=indexing
    n4 = for {
      tunnel: w12 -> [w18] mode=indexing
      tunnel: w11 -> [w16] mode=indexing
      tunnel: [w13] -> w10 mode=indexing
      n5 = Concatenate Strings(w18, "/" ("string")) -> (w15:string)
      n6 = Search and Replace String(replace all?=TRUE ("replace all? (F)"), input string=w16, search string=w15) -> (result string=w13:string)  [unwired: 5 in, 3 out]
    }
  }
  n7 = Insert Into Array(array=w4, index (col)=0 ("disabled index (col)"), new element=w2) -> (→"Route Specs":string[][])  [unwired: 1 in]
